vi "Queue initial.vi"(8 "Error in (no error)":errorcluster caption="error out（no error）") -> (0 "Error out":errorcluster caption="error out", 3 "Queue output":refnum<queue>)   [LabVIEW 2011]
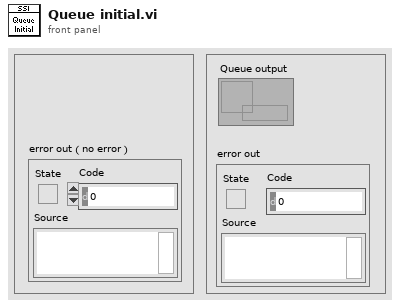
[diagram p1: front panel]
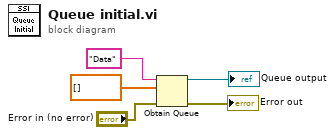
[diagram p0: block diagram]
diagram:
  n1 = Obtain Queue(name (unnamed)="Data" ("名称（未命名）"), element data type=sgl[] [], error in (no error)="Error in (no error)") -> (queue out=→"Queue output":refnum<queue>, error out=→"Error out":errorcluster)  [unwired: 2 in, 1 out]
